vi "Graph Data.vi"(8 "error in (no error)":errorcluster, 11 "Generador de Funciones in":refnum<class "Generador de Funciones.lvclass">) -> (0 "error out":errorcluster, 3 "Generador de Funciones out":refnum<class "Generador de Funciones.lvclass">)   [LabVIEW 2020, in "Generador de Funciones.lvlib" / "Generador de Funciones.lvclass"]
uses:
  Generador de Funciones.lvclass
  Generador de Funciones.lvclass/Generador de Funciones.ctl
  Logging Txt/Logging Txt Messages/Save data Msg/Save data Msg.lvclass/Save data Msg.ctl
  <vilib>/ActorFramework/Message Enqueuer/Message Enqueuer.lvclass/Message Enqueuer.ctl
  <vilib>/ActorFramework/Message Enqueuer/Enqueue.vi
  Logging Txt/Logging Txt Messages/Save data Msg/Save data Msg.lvclass
  C:/Program Files (x86)/National Instruments/LabVIEW 2020/vi.lib/ActorFramework/Message/Message.lvclass
  <vilib>/ActorFramework/Message Priority Queue/Priority Enqueue.vi
  <vilib>/measure/NI_MABase.lvlib
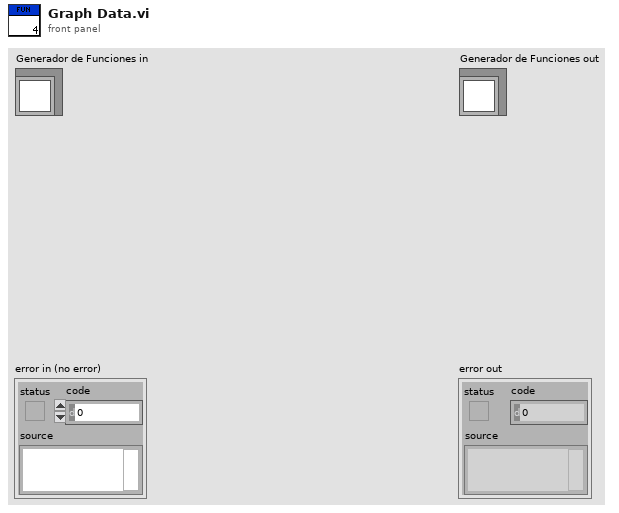
[diagram p1: front panel]
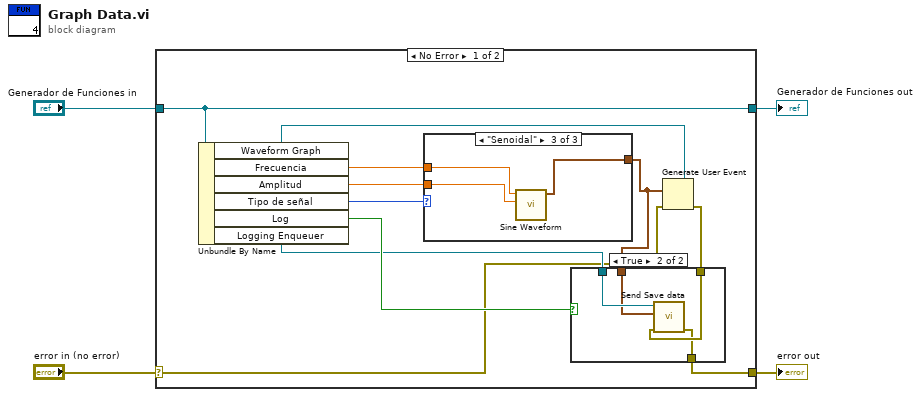
[diagram p0: block diagram]
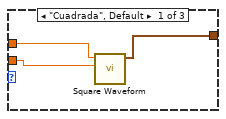
[diagram p3: hidden frame]
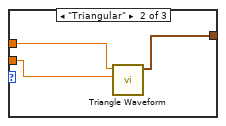
[diagram p4: hidden frame]
diagram:
  n1 = case shown="No Error" "error in (no error)" {
    selector: "error in (no error)" -> [w6 w31]
    tunnel: [w5 w31] -> w3
    tunnel: [w12 w30] -> w1
    tunnel: "Generador de Funciones in" -> [w12 w30]
    frame No Error {
      n2 = Unbundle By Name(w12) -> ("Waveform Graph"=w11:refnum<user-event>, "Frecuencia"=w14:dbl, "Amplitud"=w13:dbl, "Tipo de señal"=w15:enum16{"Cuadrada", "Triangular", "Senoidal"}, "Log"=w10:bool, "Logging Enqueuer"=w9:refnum<class "Message Enqueuer.lvclass">)
      n3 = case shown="\"Senoidal\"" w15 {
        tunnel: w14 -> [w22 w26 w29]
        tunnel: w13 -> [w21 w25 w28]
        tunnel: [w23 w24 w27] -> w8
        frame "Cuadrada", Default {
          n4 = call <vilib>:"Square Waveform.vi"("amplitude"=w21, "frequency"=w22) -> ("signal out"=w23:waveform(dbl))  [unwired: 8 in, 1 out]
        }
        frame "Triangular" {
          n5 = call <vilib>:"Triangle Waveform.vi"("amplitude"=w25, "frequency"=w26) -> ("signal out"=w24:waveform(dbl))  [unwired: 8 in, 1 out]
        }
        frame "Senoidal" {
          n6 = call <vilib>:"Sine Waveform.vi"("amplitude"=w28, "frequency"=w29) -> ("signal out"=w27:waveform(dbl))  [unwired: 8 in, 1 out]
        }
      }
      n7 = Generate User Event(user event=w11, event data cluster=w8, error in=w6) -> (error out=w7:errorcluster)  [unwired: 1 in, 1 out]
      n8 = case shown="True" w10 {
        tunnel: w9 -> [_ w20]
        tunnel: w8 -> [_ w19]
        tunnel: w7 -> [w16 w18]
        tunnel: [w16 w17] -> w5
        frame False {
        }
        frame True {
          n9 = call "Send Save data.vi"("error in (no error)"=w18, "signal out"=w19, "Message Enqueuer"=w20) -> ("error out"=w17:errorcluster)  [unwired: 7 in, 1 out]
        }
      }
    }
    frame Error {
    }
  }
  "error out" <- w3
  "Generador de Funciones out" <- w1
